vi "MGI ERD Base Storage FG.vi"(9 "error[]":errorcluster[](array[cluster]), 11 "MGI Error Reporter Dialog in":refnum<class "MGI Error Reporter Dialog.lvclass">) -> (2 "LB Row Inserted[]":i32[](array[numeric]), 3 "MGI Error Reporter Dialog Out":refnum<class "MGI Error Reporter Dialog.lvclass">)   [LabVIEW 2020, in "MGI Error Reporter Dialog.lvclass"]
doc: "This factory VI processes the error[] specified and adds MGI ERD Storage classes to the specified array as necessary. This VI must maintain the MGI ERD Storage[] order, which should match the order it appears in the listbox.\nRecent errors are added at the top of the Error History listbox.\n\nAuthored by Shawn Walpole\nsupport@mooregoodideas.com\nwww.mooregoodideas.com\n\nCopyright (c) 2010, Moore Good Ideas, Inc.\n\nAll rights reserved.\n\nRedistribution and use in source and binary forms, with or without modification, are permitted provided that the following conditions are met:\n\n * Redistributions of source code must retain the above copyright notice, this list of conditions and the following disclaimer.\n * Redistributions in binary form must reproduce the above copyright notice, this list of conditions and the following disclaimer in the documentation and/or other materials provided with the distribution.\n * Neither the name of Moore Good Ideas, Inc. nor the names of its contributors may be used to endorse or promote products derived from this software without specific prior written permission.\n\nTHIS SOFTWARE IS PROVIDED BY THE COPYRIGHT HOLDERS AND CONTRIBUTORS \"AS IS\" AND ANY EXPRESS OR IMPLIED WARRANTIES, INCLUDING, BUT NOT LIMITED TO, THE IMPLIED WARRANTIES OF MERCHANTABILITY AND FITNESS FOR A PARTICULAR PURPOSE ARE DISCLAIMED. IN NO EVENT SHALL THE COPYRIGHT OWNER OR CONTRIBUTORS BE LIABLE FOR ANY DIRECT, INDIRECT, INCIDENTAL, SPECIAL, EXEMPLARY, OR CONSEQUENTIAL DAMAGES (INCLUDING, BUT NOT LIMITED TO, PROCUREMENT OF SUBSTITUTE GOODS OR SERVICES; LOSS OF USE, DATA, OR PROFITS; OR BUSINESS INTERRUPTION) HOWEVER CAUSED AND ON ANY THEORY OF LIABILITY, WHETHER IN CONTRACT, STRICT LIABILITY, OR TORT (INCLUDING NEGLIGENCE OR OTHERWISE) ARISING IN ANY WAY OUT OF THE USE OF THIS SOFTWARE, EVEN IF ADVISED OF THE POSSIBILITY OF SUCH DAMAGE."
uses:
  <userlib>/_MGI/Error Reporter/MGI Error Reporter Dialog/MGI Error Reporter Dialog.lvclass
  <userlib>/_MGI/Error Reporter/MGI Error Reporter Dialog/MGI ERD LB Row Base/MGI ERD LB Row Base.lvclass
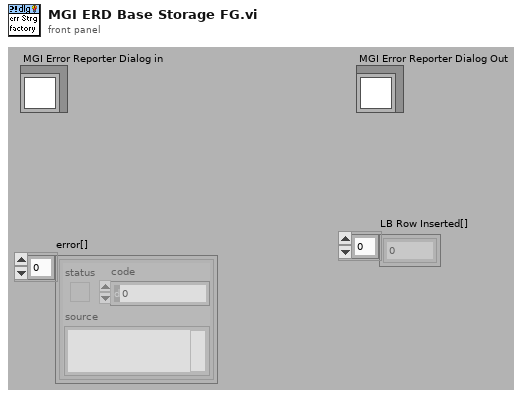
[diagram p1: front panel]
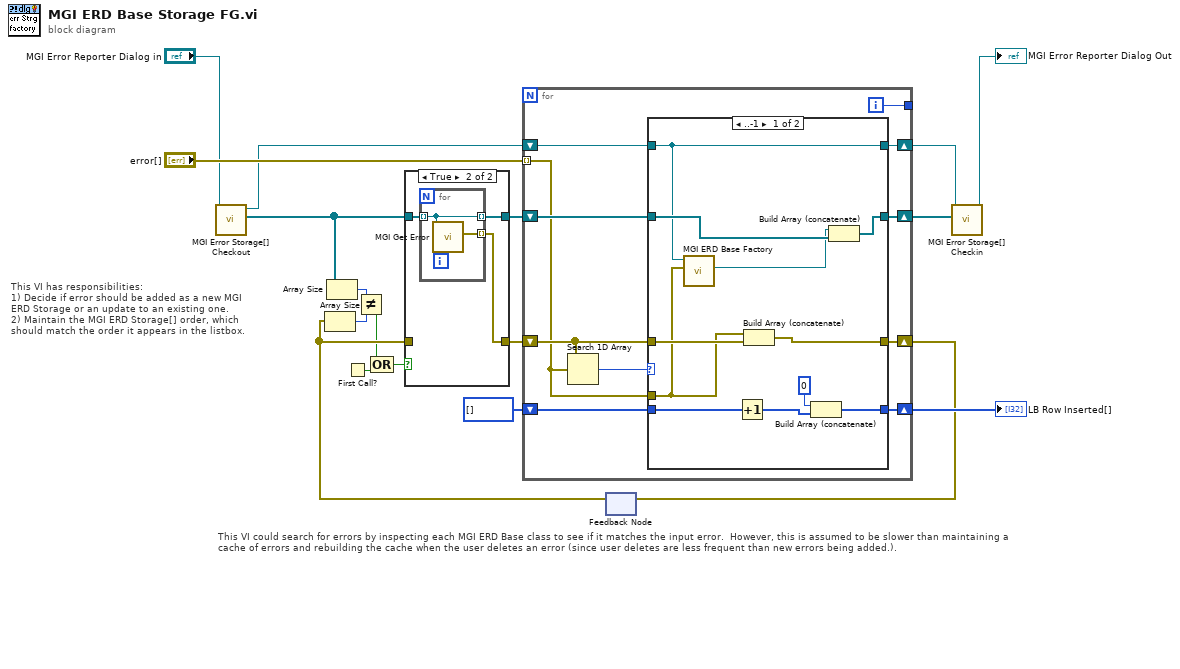
[diagram p0: block diagram]
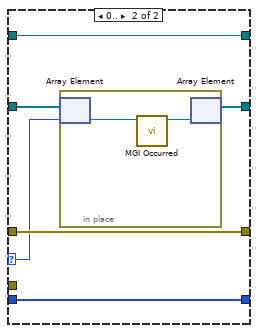
[diagram p2: hidden frame]
diagram:
  # "This VI has responsibilities:\n1) Decide if error should be added as a new MGI ERD Storage or an update to an existing one.\n2) Maintain the MGI ERD Storage[] order, which should match the order it appears in the listbox."
  # "This VI could search for errors by inspecting each MGI ERD Base class to see if it matches the input error.  However, this is assumed to be slower than maintaining a cache of errors and rebuilding the cache when the user deletes an error (since user deletes are less frequent than new errors being added.)."
  n1 = call <userlib>:"MGI Error Storage[] Checkout.vi"("MGI Error Reporter Dialog In"="MGI Error Reporter Dialog in") -> ("ErrStorage[row]"=w17:refnum<class "MGI ERD LB Row Base.lvclass">[], "MGI Error Reporter Dialog Out"=w2:refnum<class "MGI Error Reporter Dialog.lvclass">)  [unwired: 9 out]
  n2 = Array Size(array=w17) -> (size(s)=w8:i32)
  n3 = First Call?() -> (First Call?: T/F=w10:bool)
  n4 = feedback #1() -> (w11:errorcluster[])  [unwired: 1 out]
  n5 = Array Size(array=w11) -> (size(s)=w7:i32)
  n6 = Not Equal?(x=w8, y=w7) -> (x != y?=w6:bool)
  n7 = Compound Arithmetic op=OR(w6, w10) -> (w9:bool)
  n8 = case shown="True" w9 {
    tunnel: w11 -> [w19 _]
    tunnel: w17 -> [w20 w23]
    tunnel: [w20 w22] -> w4
    tunnel: [w19 w21] -> w5
    frame False {
    }
    frame True {
      n9 = for {
        tunnel: w23 -> [w25] mode=indexing
        tunnel: [w25] -> w22 mode=indexing
        tunnel: [w24] -> w21 mode=indexing
        n10 = call <userlib>:"MGI Get Error.vi"("MGI ERD LB Row Base in"=w25) -> ("error"=w24:errorcluster)  [unwired: 10 out]
      }
    }
  }
  n11 = for {
    shift-right: [w35] -> w12
    shift-left: w5 -> [w31]
    shift-right: [w33] -> w16
    shift-left: w4 -> [w36]
    tunnel: "error[]" -> [w30] mode=indexing
    tunnel: [w34] -> _
    shift-right: [w29] -> w13
    shift-left: i32[] [] -> [w28]
    shift-right: [w26] -> w1
    shift-left: w2 -> [w27]
    i -> [w34]
    n12 = Search 1D Array(1D array=w31, element=w30) -> (index of element=w32:i32)  [unwired: 1 out]
    n13 = case shown="..-1" w32 {
      selector: w32 -> [_ w50]
      tunnel: w36 -> [w47 w51]
      tunnel: w31 -> [w45 w53]
      tunnel: [w44 w53] -> w35
      tunnel: [w46 w49] -> w33
      tunnel: w30 -> [w39 _]
      tunnel: [w42 w52] -> w29
      tunnel: w28 -> [w41 w52]
      tunnel: w27 -> [w38 w48]
      tunnel: [w38 w48] -> w26
      frame ..-1 {
        n14 = call-dynamic "MGI ERD Base Factory.vi"("error"=w39, "MGI Error Reporter Dialog in"=w38) -> ("MGI ERD LB Row Base"=w37:refnum<class "MGI ERD LB Row Base.lvclass">)  [unwired: 9 out]
        n15 = Increment(x=w41) -> (x+1=w40:i32[])
        n16 = Build Array (concatenate)(w39, w45) -> (w44:errorcluster[])
        n17 = Build Array (concatenate)(0, w40) -> (w42:i32[])
        n18 = Build Array (concatenate)(w37, w47) -> (w46:refnum<class "MGI ERD LB Row Base.lvclass">[])
      }
      frame 0.. {
        n19 = in-place {
          n20 = in-place-array #2(w51, w50) -> (w54:refnum<class "MGI ERD LB Row Base.lvclass">)
          n21 = call-dynamic "MGI Occurred.vi"("MGI ERD LB Row Base in"=w54) -> ("MGI ERD LB Row Base out"=w55:refnum<class "MGI ERD LB Row Base.lvclass">)  [unwired: 10 out]
          n22 = in-place-array #2(w55) -> (w49:refnum<class "MGI ERD LB Row Base.lvclass">[])  [unwired: 1 out]
        }
      }
    }
  }
  "LB Row Inserted[]" <- w13
  n23 = feedback-in #1(w12) -> ()
  n24 = call <userlib>:"MGI Error Storage[] Checkin.vi"("ErrStorage[row]"=w16, "MGI Error Reporter Dialog In"=w1) -> ("MGI Error Reporter Dialog Out"=→"MGI Error Reporter Dialog Out":refnum<class "MGI Error Reporter Dialog.lvclass">)  [unwired: 9 out]
